vi "SubVI_PrePolarisation.vi"(0 "Test References":T3, 1 "Polar Params SubVIv2":T2, 2 "Scan Polar Params":refnum<vi>[](array[refnum])) -> ()   [LabVIEW 2019]
uses:
  TypeDefs/AcqMode.ctl
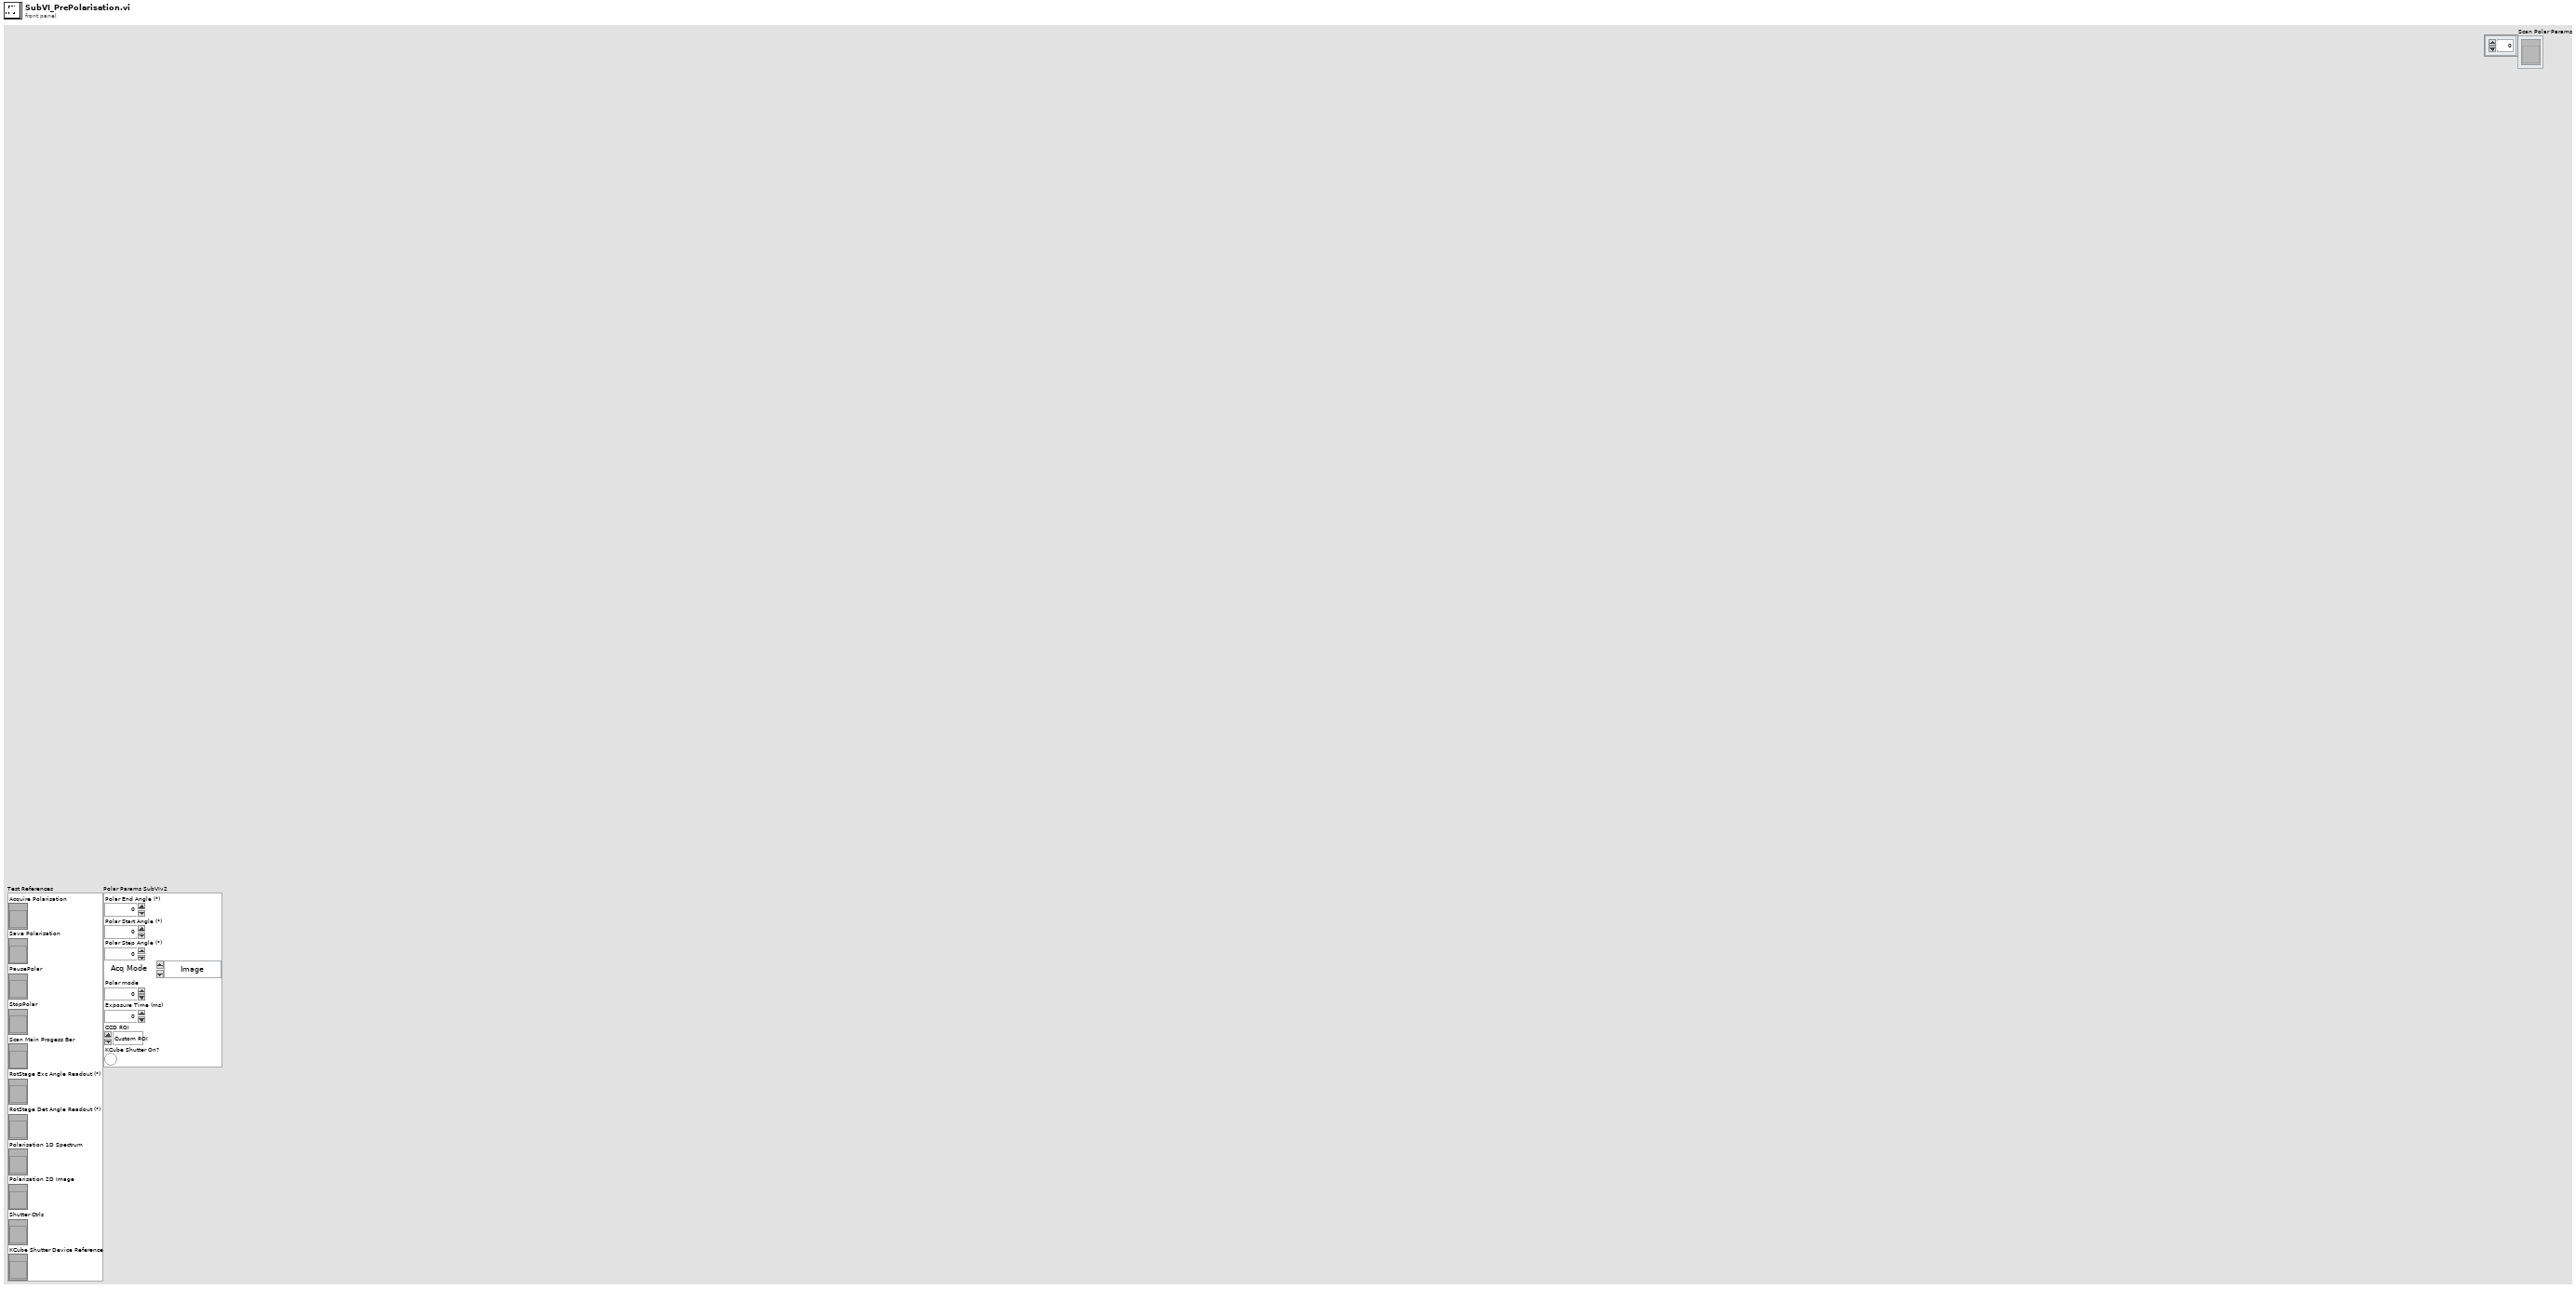
[diagram p1: front panel]
types:
  T1 = typedef "AcqMode.ctl" = enum16{"Image", "Spectrum", "APD 1", "APD 2", "APD 1+2"}
  T2 = cluster{"Polar End Angle (°)":dbl, "Polar Start Angle (°)":dbl, "Polar Step Angle (°)":dbl, "Acq Mode":T1, "Polar mode":u16, "Exposure Time (ms)":dbl, "CCD ROI":enum16{"Custom ROI", "Full sensor", "Binned full sensor"}, "KCube Shutter On?":bool}
  T3 = cluster{"Acquire Polarisation":refnum<vi>, "Save Polarisation":refnum<vi>, "PausePolar":refnum<vi>, "StopPolar":refnum<vi>, "Scan Main Progess Bar":refnum<vi>, "RotStage Exc Angle Readout (°)":refnum<vi>, "RotStage Det Angle Readout (°)":refnum<vi>, "Polarisation 1D Spectrum":refnum<vi>, "Polarisation 2D Image":refnum<vi>, "Shutter Ctrls":refnum<vi>, "KCube Shutter Device Reference":refnum<vi>}
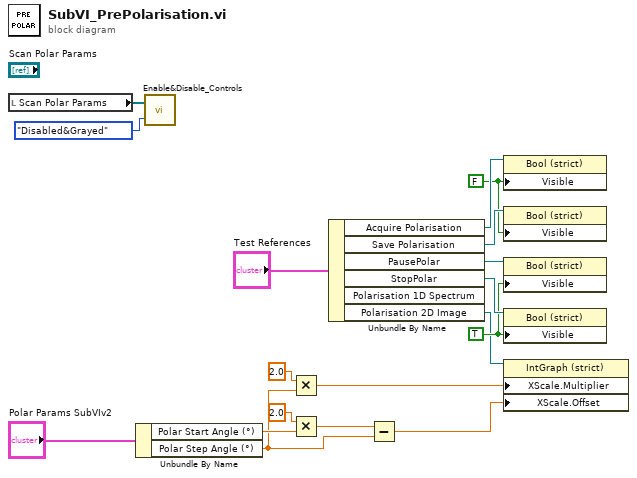
[diagram p0: block diagram]
diagram:
  w11 = TRUE ("Visible")
  w12 = FALSE ("Visible")
  n1 = local read "Scan Polar Params"() -> (w10:refnum<vi>[])
  n2 = Unbundle By Name("Polar Params SubVIv2") -> ("Polar Start Angle (°)"=w4:dbl, "Polar Step Angle (°)"=w2:dbl)
  n3 = call "Enable&Disable_Controls.vi"("Enum"=enum16{"Enabled", "Disabled", "Disabled&Grayed"}."Disabled&Grayed", "References"=w10) -> ()  [unwired: 1 in]
  n4 = Multiply(x=2.0, y=w2) -> (x*y=w6:dbl)
  n5 = Multiply(x=2.0, y=w4) -> (x*y=w3:dbl)
  n6 = Unbundle By Name("Test References") -> ("Acquire Polarisation"=w16:refnum<vi>, "Save Polarisation"=w15:refnum<vi>, "PausePolar"=w14:refnum<vi>, "StopPolar"=w13:refnum<vi>, "Polarisation 2D Image"=w8:refnum<vi>)  [unwired: 1 out]
  n7 = Subtract(x=w3, y=w2) -> (x-y=w1:dbl)
  n8 = property class="Bool (strict)"(reference=w16, "Visible"=w12) -> ()  [unwired: 1 in, 2 out]
  n9 = property class="Bool (strict)"(reference=w15, "Visible"=w12) -> ()  [unwired: 1 in, 2 out]
  n10 = property class="Bool (strict)"(reference=w14, "Visible"=w11) -> ()  [unwired: 1 in, 2 out]
  n11 = property class="Bool (strict)"(reference=w13, "Visible"=w11) -> ()  [unwired: 1 in, 2 out]
  n12 = property class="IntGraph (strict)"(reference=w8, "XScale.Multiplier"=w6, "XScale.Offset"=w1) -> ()  [unwired: 1 in, 2 out]
